vi "Instrument Error Lookup.vi"(11 "Error Code (00)":string="00") -> (3 "Error Message":string)   [LabVIEW 2015, in "Fluke 28x Series.lvlib"]
doc: "This VI uses the instrument-provided error code to output the respective error message."
uses:
  <instrlib>/Fluke 28x Series/Fluke 28x Series.lvlib
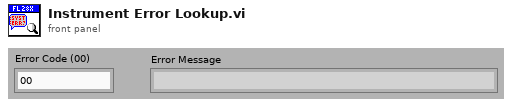
[diagram p1: front panel]
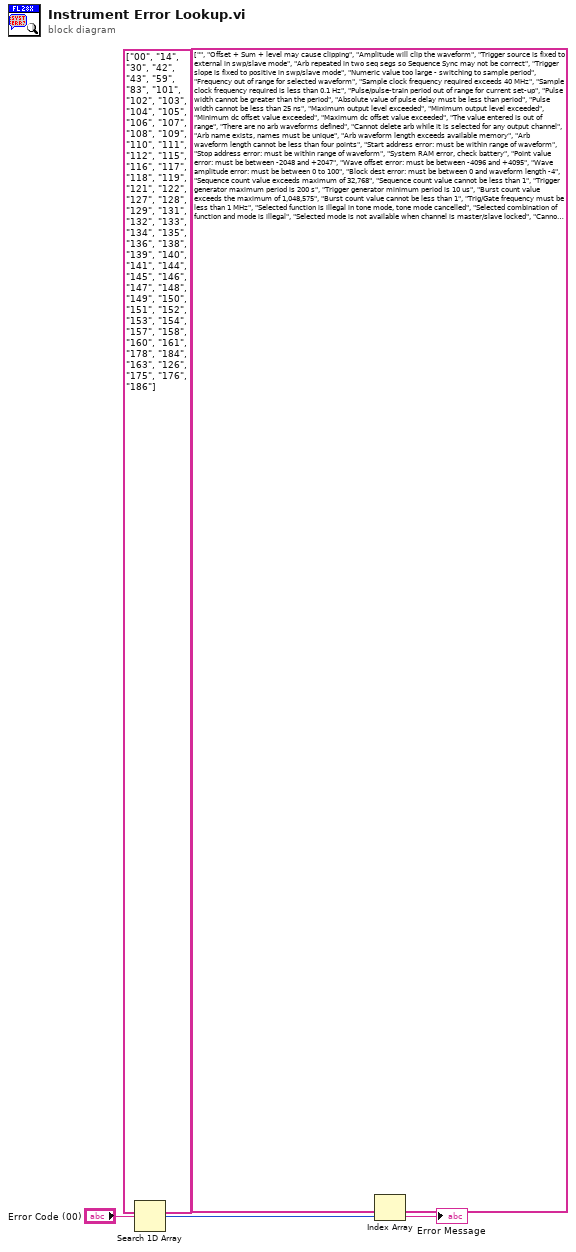
[diagram p0: block diagram]
diagram:
  n1 = Search 1D Array(1D array=string[] ["00", "14", "30", "42", "43", "59", "83", "101", "102", "103", "104", "105", "106", "107", "108", "109", "110", "111", "112", "115", "116", "117", "118", "119", "121", "122", "127", "128", "129", "131", "132", "133", "134", "135", "136", "138", "139", "140", "141", "144", "145", "146", "147", "148", "149", "150", "151", "152", "153", "154", "157", "158", "160", "161", "178", "184", "163", "126", "175", "176", "186"], element="Error Code (00)") -> (index of element=w5:i32)  [unwired: 1 in]
  n2 = Index Array(array=string[] ["", "Offset + Sum + level may cause clipping", "Amplitude will clip the waveform", "Trigger source is fixed to external in swp/slave mode", "Arb repeated in two seq segs so Sequence Sync may not be correct", "Trigger slope is fixed to positive in swp/slave mode", "Numeric value too large - switching to sample period", "Frequency out of range for selected waveform", "Sample clock frequency required exceeds 40 MHz", "Sample clock frequency required is less than 0.1 Hz", "Pulse/pulse-train period out of range for current set-up", "Pulse width cannot be greater than the period", "Absolute value of pulse delay must be less than period", "Pulse width cannot be less than 25 ns", "Maximum output level exceeded", "Minimum output level exceeded", "Minimum dc offset value exceeded", "Maximum dc offset value exceeded", "The value entered is out of range", "There are no arb waveforms defined", "Cannot delete arb while it is selected for any output channel", "Arb name exists, names must be unique", "Arb waveform length exceeds available memory", "Arb waveform length cannot be less than four points", "Start address error: must be within range of waveform", "Stop address error: must be within range of waveform", "System RAM error, check battery", "Point value error: must be between -2048 and +2047", "Wave offset error: must be between -4096 and +4095", "Wave amplitude error: must be between 0 to 100", "Block dest error: must be between 0 and waveform length -4", "Sequence count value exceeds maximum of 32,768", "Sequence count value cannot be less than 1", "Trigger generator maximum period is 200 s", "Trigger generator minimum period is 10 us", "Burst count value exceeds the maximum of 1,048,575", "Burst count value cannot be less than 1", "Trig/Gate frequency must be less than 1 MHz", "Selected function is illegal in tone mode, tone mode cancelled", "Selected combination of function and mode is illegal", "Selected mode is not available when channel is master/slave locked", "Cannot delete arbitrary waveforms when sequence is running", "Current set up requires an arbitrary waveform which does not exist", "Trig/gate mode and sequence step value cause a trigger conflict", "Sequence step value cannot mix edge and level between segments", "Number of pulses in train must be between 1 and 10", "Pulse train offset must be between -5.0 and +5.0 volts", "Pulse level must be between -5.0 and +5.0 volts", "Pulse number must be between 1 and 10", "Sweep frequency values must be 0.001 mHz to 1 MHz ", "Sweep time value is out of range, 0.03 to 99.9 seconds", "Sweep marker value is out of range, 0.001 Hz to 16 MHz", "Phase locking operation has failed", "Illegal phase value", "SUM ratio not possible within level constraints", "SUM or modulation conflict", "Specified arbitrary waveform name does not exist", "Illegal store number requested", "Cannot insert arbitrary waveform into itself", "Pattern value is illegal or pattern is too long", "Inter channel lock not possible. Refer to manual for more details. "], index=w5) -> (element=→"Error Message":string)
